vi "Operator Joystick.vi"(9 "Buttons":bool[](array[boolean]), 10 "Axes":dbl[](array[numeric])) -> ()   [LabVIEW 2018]
panel:
  out "Intake Wrist":T1(ring)=enum."Reverse Cargo"
  out "Elevator Level":T2(ring)
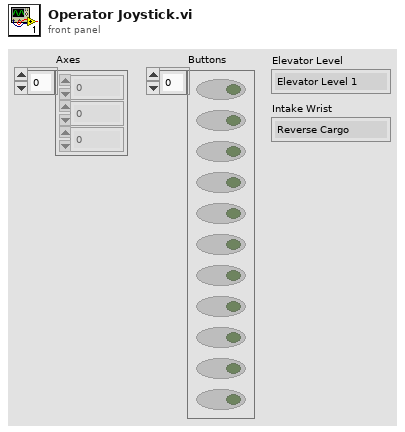
[diagram p1: front panel]
types:
  T1 = enum16{"Intake Cargo", "Outtake Cargo", "Reverse Cargo", "Intake Hatches", "Outtake Hatches"}
  T2 = enum16{"Elevator Level 1", "Elevator Level 2", "Elevator Level 3"}
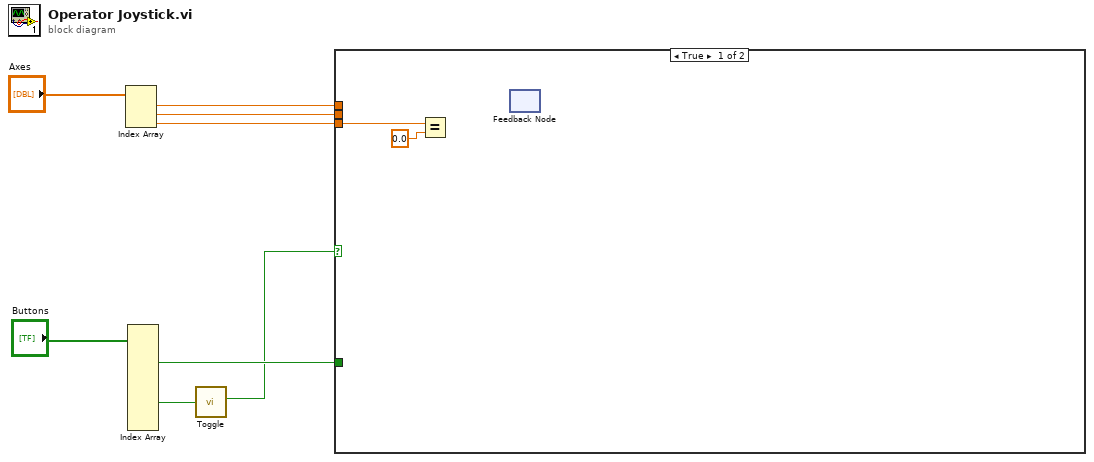
[diagram p0: block diagram]
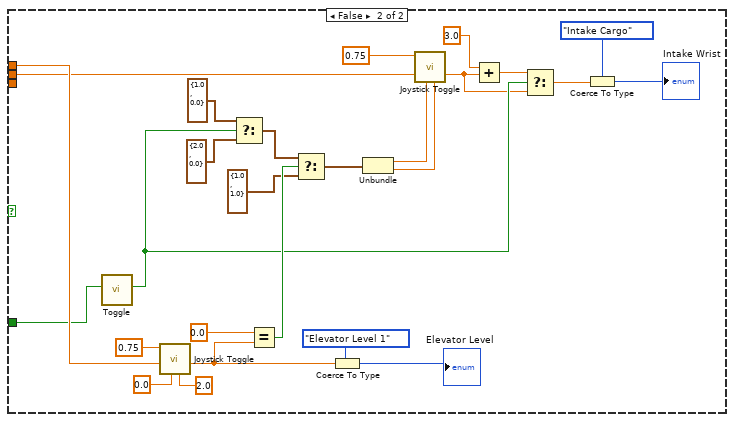
[diagram p2: hidden frame]
diagram:
  n1 = Index Array(array="Axes") -> (element #1=w6:dbl, element #2=w4:dbl, element #3=w1:dbl)  [unwired: 3 in]
  n2 = Index Array(array="Buttons") -> (element #3=w5:bool, element #8=w3:bool)  [unwired: 11 in, 9 out]
  n3 = call "Toggle.vi"("Input"=w3) -> ("Output"=w2:bool)  [unwired: 10 in]
  n4 = case shown="True" w2 {
    tunnel: w6 -> [_ w32]
    tunnel: w5 -> [_ w26]
    tunnel: w4 -> [_ w11]
    tunnel: w1 -> [w10 _]
    frame True {
      n5 = Equal?(x=w10, y=0.0) -> ()  [unwired: 1 out]
      n6 = feedback-in #1() -> ()  [unwired: 1 out]
      n7 = feedback #1() -> ()  [unwired: 2 in]
    }
    frame False {
      n8 = call "Toggle.vi"("Input"=w26) -> ("Output"=w16:bool)  [unwired: 10 in]
      n9 = call "Joystick Toggle.vi"("Max"=2.0, "Min"=0.0, "Value"=w32, "Range"=0.75) -> ("Output"=w28:dbl)  [unwired: 7 in]
      n10 = Select(t=cluster{"Range":dbl, "Range 2":dbl} {"Range"=1.0, "Range 2"=0.0}, s=w16, f=cluster{"Range":dbl, "Range 2":dbl} {"Range"=2.0, "Range 2"=0.0}) -> (s? t:f=w20:cluster{"Range":dbl, "Range 2":dbl})
      n11 = Equal?(x=0.0, y=w28) -> (x = y?=w19:bool)
      n12 = Select(t=w20, s=w19, f=cluster{"Range":dbl, "Range 2":dbl} {"Range"=1.0, "Range 2"=1.0}) -> (s? t:f=w21:cluster{"Range":dbl, "Range 2":dbl})
      n13 = Coerce To Type(0:w28, 1:T2."Elevator Level 1") -> (2:→"Elevator Level":T2)
      n14 = Unbundle(w21) -> ("Range"=w23:dbl, "Range 2"=w22:dbl)
      n15 = call "Joystick Toggle.vi"("Max"=w22, "Min"=w23, "Value"=w11, "Range"=0.75) -> ("Output"=w12:dbl)  [unwired: 7 in]
      n16 = Add(x=3.0 ("y"), y=w12) -> (x+y=w13:dbl)
      n17 = Select(t=w13, s=w16, f=w12) -> (s? t:f=w17:dbl)
      n18 = Coerce To Type(0:w17, 1:T1."Intake Cargo") -> (2:→"Intake Wrist":T1)
    }
  }
